vi "Init.vi"(8 "error in (no error)":errorcluster, 9 "SA Pin":string, 10 "Measurement Name":string) -> (0 "error out":errorcluster, 3 "TDSCDMA_OBW out":refnum<class "TDSCDMA_OBW.lvclass">)   [LabVIEW 2016, in "SeqAuto Evaluations.lvlib" / "TDSCDMA_OBW.lvclass"]
uses:
  TDSCDMA_OBW.lvclass
  C:/Sequence Automation/Plugins/SeqAuto IEvaluation.lvlibp/SeqAuto IEvaluation.lvclass
  Plugins/SeqAuto IEvaluation.lvlibp/Write Measurement Name.vi
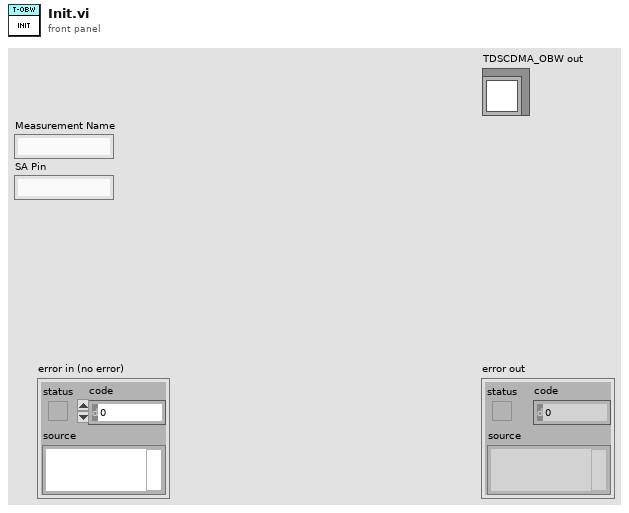
[diagram p1: front panel]
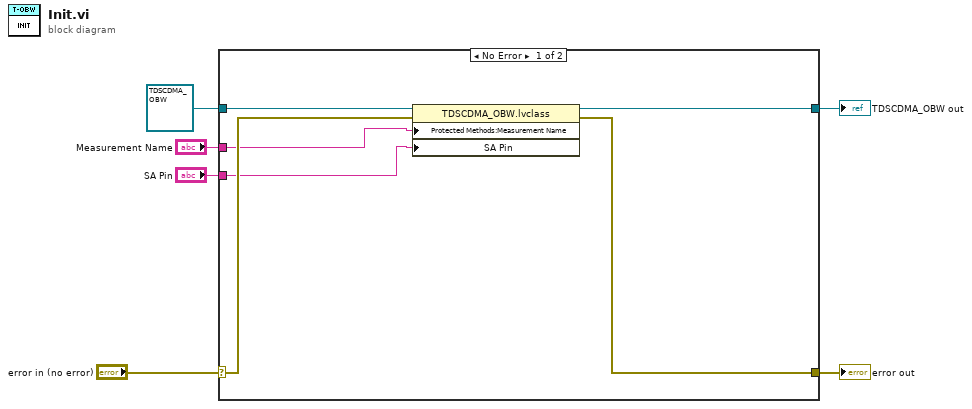
[diagram p0: block diagram]
diagram:
  n1 = case shown="No Error" "error in (no error)" {
    selector: "error in (no error)" -> [w12 w14]
    tunnel: [w11 w14] -> w5
    tunnel: [w9 w13] -> w3
    tunnel: refnum<class "TDSCDMA_OBW.lvclass"> refnum ("TDSCDMA_OBW in") -> [w10 w13]
    tunnel: "Measurement Name" -> [w8 _]
    tunnel: "SA Pin" -> [w7 _]
    frame No Error {
      n2 = property class="TDSCDMA_OBW.lvclass"(reference=w10, error in=w12, "Protected Methods:Measurement Name"=w8, "SA Pin"=w7) -> (reference out=w9:refnum<class "TDSCDMA_OBW.lvclass">, error out=w11:errorcluster)
    }
    frame Error {
    }
  }
  "error out" <- w5
  "TDSCDMA_OBW out" <- w3
